vi "Write Error Handler Interface.vi"(8 "error in (no error)":errorcluster, 10 "Error Handler Interface":refnum<class "Error Handler Interface.lvclass">, 11 "Error Handler Interface Test in":refnum<class "Error Handler Interface Test.lvclass">) -> (0 "error out":errorcluster, 3 "Error Handler Interface Test out":refnum<class "Error Handler Interface Test.lvclass">)   [LabVIEW 2020, in "Error Handler Interface Test.lvclass"]
uses:
  Error Handler Interface Test.lvclass
  Framework/Error Handler Interface/Error Handler Interface.lvclass
  Error Handler Interface Test.lvclass/Error Handler Interface Test.ctl
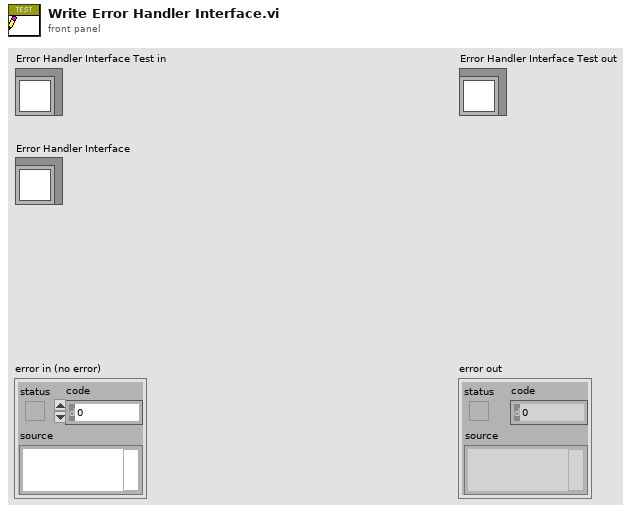
[diagram p1: front panel]
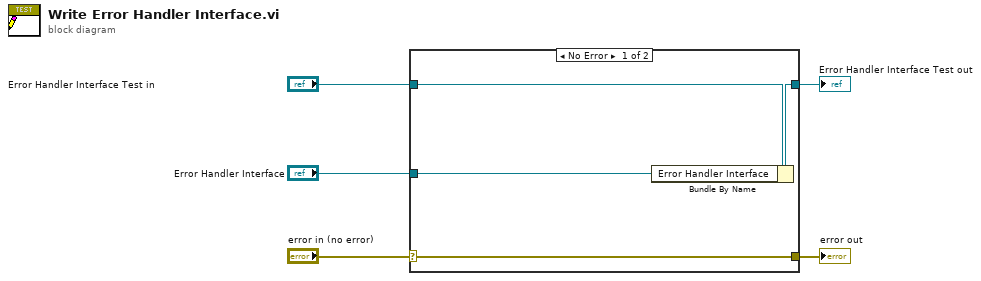
[diagram p0: block diagram]
diagram:
  n1 = case shown="No Error" "error in (no error)" {
    selector: "error in (no error)" -> [w9 w10]
    tunnel: [w9 w10] -> w4
    tunnel: [w7 w11] -> w2
    tunnel: "Error Handler Interface Test in" -> [w8 w11]
    tunnel: "Error Handler Interface" -> [w6 _]
    frame No Error {
      n2 = Bundle By Name(cluster=w8, "Error Handler Interface"=w6) -> (w7:refnum<class "Error Handler Interface Test.lvclass">)
    }
    frame Error {
    }
  }
  "error out" <- w4
  "Error Handler Interface Test out" <- w2
